vi "1-1.vi"() -> ()   [LabVIEW 2018]
panel:
  out "i值":dbl
  in  "循环次数":i8
  out "输出值":dbl
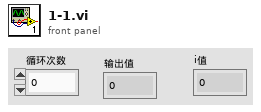
[diagram p1: front panel]
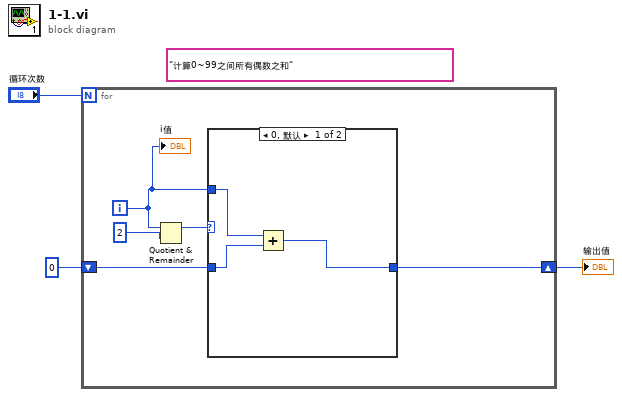
[diagram p0: block diagram]
diagram:
  (unwired) "计算0~99之间所有偶数之和"
  n1 = for {
    N: "循环次数" -> [_]
    shift-right: [w6] -> w1
    shift-left: 0 -> [w7]
    i -> [w4]
    n2 = Quotient & Remainder(x=w4, y=2) -> (x-y*floor(x/y)=w5:i32)  [unwired: 1 out]
    n3 = case shown="0, 默认" w5 {
      tunnel: w7 -> [w11 w12]
      tunnel: w4 -> [w10 _]
      tunnel: [w9 w12] -> w6
      frame 0, Default {
        n4 = Add(x=w10, y=w11) -> (x+y=w9:i32)
      }
      frame 1 {
      }
    }
    "i值" <- w4
  }
  "输出值" <- w1
